vi "ToWarning.vi"(9 "Error in":errorcluster) -> (1 "Warning out":errorcluster)   [LabVIEW 2017, in "GPError.lvlib"]
doc: "If there is an error on <B>Error in</B> this VI converts it to a warning and returns it on <B>Warning out</B>. If no error is on <B>Error in</B>, this VI doesn't change the error wire.\n\nThis VI supports appended errors, converting all errors to warnings.\n\nThis VI is inlined.\n\nSteen Schmidt\nGPower\n18/7 2013"
uses:
  GPError.lvlib
  Append/AppendMulti.vi
panel:
  # "Copyright © 2013\nSteen Schmidt, GPower\nSee enclosed license file for terms and conditions"
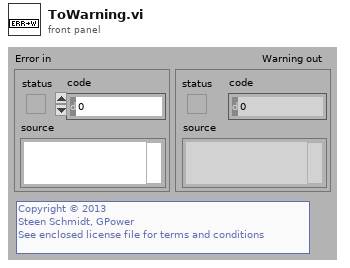
[diagram p1: front panel]
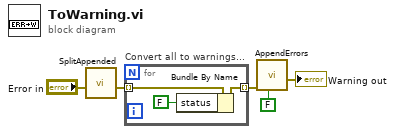
[diagram p0: block diagram]
diagram:
  n1 = call "SplitAppended.vi"("Appended errors in"="Error in") -> ("Errors out"=w4:errorcluster[])  [unwired: 10 in]
  n2 = for "Convert all to warnings..." {
    tunnel: w4 -> [w8] mode=indexing
    tunnel: [w7] -> w2 mode=indexing
    n3 = Bundle By Name(cluster=w8, "status"=FALSE) -> (w7:errorcluster)
  }
  n4 = call-poly "AppendErrors.vi"("Only append if new?"=FALSE, "Errors to append"=w2) -> ("Appended errors out"=→"Warning out":errorcluster)  [unwired: 9 in]
